vi "VerifyStopBytes.vi"(7 "Index":i32, 8 "Data Buffer":u8[](array[numeric]) format="%.0x") -> (2 "Found":bool)   [LabVIEW 2010]
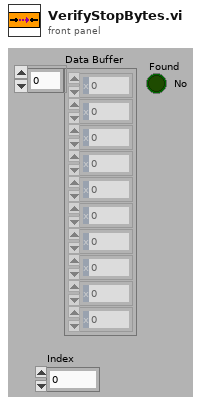
[diagram p1: front panel]
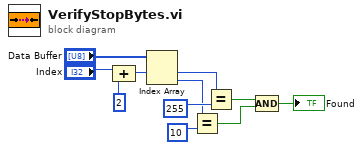
[diagram p0: block diagram]
diagram:
  n1 = Compound Arithmetic op=ADD("Index", 2 ("value")) -> (w3:i32)
  n2 = Index Array(array="Data Buffer", index #1=w3) -> (element #1=w11:u8, element #2=w7:u8)  [unwired: 1 in]
  n3 = Equal?(x=w7, y=u8 10) -> (x = y?=w5:bool)
  n4 = Equal?(x=w11, y=u8 255) -> (x = y?=w6:bool)
  n5 = Compound Arithmetic op=AND(w6, w5) -> (→"Found":bool)
